vi "UHR-Fleezers Control (host) - 16.2.2v2.vi"() -> ()   [LabVIEW 2014] (continued)
                    n1840 = property on="Red Laser ON" class="Bool (strict)"("Val(Sgnl)"=TRUE ("Value (Signaling)")) -> ()  [unwired: 2 in, 2 out]
                  }
                }
              }
              frame #3 {
                n1841 = node-c288() -> (w2681:T28)  [unwired: 4 in]
                n1842 = timed-loop {
                  timing: w2681 -> [_]
                  timing-out: [_] -> w2680
                  tunnel: [w2682] -> _
                  tunnel: w2679 -> [w2682]
                  stop <- "Stop assembly line" stop-if-true
                  n1843 = node-c288() -> ()  [unwired: 1 in, 1 out]
                  n1844 = local read "APD 2 Rate (Hz)"() -> (w2686:dbl)
                  n1845 = Multiply(x="Cy5 Fl.  Thresh. (kHz)", y=1000.0) -> (x*y=w2689:dbl)
                  n1846 = Greater?(x=w2686, y=w2689) -> (0:w2685:bool)
                  n1847 = And(x=w2685, y=w2682) -> (x .and. y?=w2683:bool)
                  n1848 = case shown="True" w2683 {
                    frame False {
                    }
                    frame True {
                      n1849 = property on="Green Laser ON" class="Bool (strict)"("Val(Sgnl)"=TRUE ("Value (Signaling)")) -> ()  [unwired: 2 in, 2 out]
                    }
                  }
                  n1850 = node-c288() -> ()  [unwired: 1 in, 1 out]
                }
                n1851 = node-c288(w2680) -> ()  [unwired: 1 out]
              }
              frame #4 {
                w2696 = FALSE ("Value (Signaling)")
                # "lower spot"
                n1852 = local read "Saved Stage Positions"() -> (w2700:dbl[][])
                n1853 = property on="Red Laser ON" class="Bool (strict)"("Val(Sgnl)"=w2696) -> ()  [unwired: 2 in, 2 out]
                n1854 = property on="Green Laser ON" class="Bool (strict)"("Val(Sgnl)"=w2696) -> ()  [unwired: 2 in, 2 out]
                n1855 = local write "Stage Moving"(TRUE ("Stage Moving")) -> ()
                n1856 = local write "Stop assembly line"(FALSE ("Stop assembly line")) -> ()
                n1857 = call "move to saved stage position.vi"("Stage VISA resource name in"=w2697, "Position"=3, "Saved Stage Positions"=w2700) -> ("error out"=w2699:errorcluster)  [unwired: 1 in, 1 out]
                n1858 = local write "Stage Control Serial Error"(w2699) -> ()
              }
              frame #5 {
                w2702 = FALSE ("Stage Moving")
                n1859 = local write "Stage Moving"(w2702) -> ()
                n1860 = local write "AL Running"(w2702) -> ()
                n1861 = call <vilib>:"Beep.vi"() -> ()  [unwired: 3 in, 9 out]
              }
            }
          }
        }
      }
      event "Stop All": Value Change {
        n1862 = event-data() -> ()  [unwired: 7 out]
        n1863 = local read "Stop All"() -> (w2703:bool)
      }
    }
    n1864 = node-c288() -> ()  [unwired: 2 out]
  }
  n1865 = timed-loop "Basic control parameters (all FPGA settings, other basic controls)" {
    shift-right: [w2711] -> _
    shift-left: errorcluster {"status"=FALSE, "code"=0, "source"=""} ("error out") -> [_]
    tunnel: [w2710] -> _
    timing: w85 -> [_]
    timing-out: [_] -> w84
    tunnel: w63 -> [w2709]
    tunnel: w55 -> [w2708]
    tunnel: w54 -> [w2707]
    tunnel: w53 -> [w2706]
    tunnel: w52 -> [w2705]
    tunnel: w36 -> [w2704]
    stop <- w2710 stop-if-true
    n1866 = node-c288() -> ()  [unwired: 2 out]
    n1867 = event shown="[34] \"Read Cal\": Value Change" {
      selector: _ -> [_ _ _ _ _ _ _ _ _ _ _ _ _ _ _ _ _ _ _ _ _ _ _ _ _ _ _ _ _ _ _ _ _ _ _ _ _ _ _ _ _ _ _ _ _ _ _ _ _ _ _ _ _ _ _ _ _ _ _ _ _ _ _ _ _ _ _ _ _ _ _ _ _ _ _ _ _ _ _ _]
      dyn-events: _ -> [_ _ _ _ _ _ _ _ _ _ _ _ _ _ _ _ _ _ _ _ _ _ _ _ _ _ _ _ _ _ _ _ _ _ _ _ _ _ _ _ _ _ _ _ _ _ _ _ _ _ _ _ _ _ _ _ _ _ _ _ _ _ _ _ _ _ _ _ _ _ _ _ _ _ _ _ _ _ _ _]
      timeout: _ -> [_ _ _ _ _ _ _ _ _ _ _ _ _ _ _ _ _ _ _ _ _ _ _ _ _ _ _ _ _ _ _ _ _ _ _ _ _ _ _ _ _ _ _ _ _ _ _ _ _ _ _ _ _ _ _ _ _ _ _ _ _ _ _ _ _ _ _ _ _ _ _ _ _ _ _ _ _ _ _ _]
      tunnel: [w2754 _ _ _ w2784 _ _ _ _ _ _ w2858 _ _ w2949 w2951 w2960 w2962 w3032 _ w3074 w3101 w3129 w3154 w3181 w3207 w3238 _ _ _ w3251 w3345 w3349 w3386 _ w3424 w3427 w3430 w3440 w3443 _ w3450 _ _ _ _ _ _ _ _ _ _ _ _ _ _ _ _ _ w3914 _ _ _ _ w3950 _ _ _ _ _ _ _ _ _ _ _ _ _ _ _] -> w2711
      tunnel: [_ _ _ _ _ _ _ _ _ w2843 _ _ _ _ _ _ _ _ _ _ _ _ _ _ _ _ _ _ _ _ _ _ _ _ _ _ _ _ _ _ _ _ _ _ _ _ _ _ _ _ _ _ _ _ _ _ _ _ _ _ _ _ _ _ _ _ _ _ _ _ _ _ _ _ _ _ _ _ _ _] -> w2710
      tunnel: [_ _ _ _ _ _ _ "Round T1 X" _ _ _ _ _ _ _ _ _ _ _ _ _ _ _ _ _ _ _ _ _ _ _ _ _ _ _ _ _ _ _ _ _ _ _ _ _ _ _ _ _ _ _ _ _ _ _ _ _ _ _ _ _ _ _ _ _ _ _ _ _ _ _ _ _ _ _ _ _ _ _ _] -> _
      tunnel: [_ _ _ "Adjust Scale\nto Mean" _ _ _ _ _ _ _ _ _ _ _ _ _ _ _ _ _ _ _ _ _ _ _ _ _ _ "Test ttrig" _ _ _ _ _ _ _ _ _ _ _ _ _ _ _ _ _ _ "Flush Sample" "Flush Pump 3" "Flush Pump 1" "Clear Volume" _ _ _ _ _ _ _ _ _ _ _ _ _ _ _ _ _ _ _ _ _ _ _ _ _ _ _] -> _
      tunnel: [_ _ _ _ _ _ _ _ "Round T2 X" _ "Delayed Interlace Start" _ _ _ _ _ _ _ _ _ _ _ _ _ _ _ _ _ _ _ _ _ _ _ _ _ _ _ _ _ _ _ _ _ _ _ _ _ _ _ _ _ _ _ _ _ _ _ _ _ _ _ _ _ _ _ _ _ _ _ _ _ _ _ _ _ _ _ _ _] -> _
      tunnel: w2709 -> [_ _ _ _ _ _ _ _ _ _ _ _ _ _ _ _ _ _ _ _ _ _ _ _ _ _ _ _ _ _ _ _ _ _ _ _ _ _ _ _ _ _ _ _ _ w3649 w3656 w3663 w3668 w3682 _ _ w3828 _ _ _ _ _ _ _ _ _ _ _ _ _ _ _ _ _ _ _ _ _ _ _ _ _ _ _]
      tunnel: w2708 -> [_ _ _ _ _ _ _ _ _ _ _ _ _ _ _ _ _ _ _ _ _ _ _ _ _ _ _ _ _ _ _ _ _ _ _ _ _ _ _ _ _ _ _ w3538 _ _ _ _ _ _ w3741 _ _ w3834 _ w3843 _ w3857 _ _ _ _ _ _ _ _ _ _ _ _ _ _ _ _ _ _ _ _ _ _]
      tunnel: w2707 -> [_ _ _ _ _ _ _ _ _ _ _ _ _ _ _ _ _ _ _ _ _ _ _ _ _ _ _ _ _ _ _ _ _ _ _ _ _ _ _ _ _ _ _ _ _ _ _ _ _ _ _ _ _ _ _ _ _ _ _ _ _ _ _ _ _ _ _ _ _ _ _ _ _ _ _ _ _ _ _ _]
      tunnel: w2706 -> [_ _ _ _ _ _ _ _ _ _ _ _ _ _ _ _ _ _ _ _ _ _ _ _ _ _ _ _ _ _ _ _ _ _ _ _ _ _ _ _ _ _ w3461 _ _ _ _ _ _ _ _ w3786 _ _ w3839 _ w3850 _ w3882 _ _ _ _ _ _ _ _ _ _ _ _ _ _ _ _ _ _ _ _ _]
      tunnel: w2705 -> [_ _ _ _ _ _ _ _ _ _ _ _ _ _ _ _ _ _ _ _ _ _ _ _ _ _ _ _ _ _ _ _ _ _ _ _ _ _ _ _ _ _ _ _ _ _ _ _ _ _ _ _ _ _ _ _ _ _ _ _ _ _ _ _ _ _ _ _ _ _ _ _ _ _ _ _ _ _ _ _]
      tunnel: w2704 -> [w2718 _ _ _ w2783 _ w2809 _ _ _ _ w2849 _ _ w2931 w2950 w2955 w2961 w2997 _ w3063 w3099 w3115 w3136 w3164 w3184 w3216 w3242 w3246 w3247 w3249 w3253 w3346 w3351 _ w3421 w3425 w3428 w3438 w3441 _ w3449 _ _ _ _ _ _ _ _ _ _ _ _ _ _ _ _ _ w3907 _ w3928 _ w3934 w3949 _ w3956 w3958 w3965 w3979 w3994 _ w4003 _ w4023 _ _ w4079 w4115 w4116]
      event "AI Count (ticks)", "Sets to FIFO (Traps)", "Save ave N", "FPGA Ave.", "# Samples/channel", "N sets to save", "APD Samples/FIFO Acq.": Value Change {
        # "So that if 'Save ave N' is updated, the AOD scanning code updates too."
        n1868 = event-data() -> ()  [unwired: 6 out]
        n1869 = local read "AI Count (ticks)"() -> (w2738:u16)
        n1870 = Unbundle By Name("Sets to FIFO (Traps)") -> ("Set 1"=w2722:bool, "Set 2"=w2721:bool, "Set 3"=w2720:bool)
        n1871 = Boolean To (0,1)(Boolean="Sets to FIFO (Traps)") -> (0, 1=w2746:cluster{"Set 1":i16, "Set 2":i16, "Set 3":i16})
        n1872 = xnode "Read/Write Control"("FPGA VI Reference In"=w2718, "ai count"=w2738, "Set 1"=w2722, "Set 2"=w2721, "Set 3"=w2720, "N of AI1 Int Acq Sets"="N Acq Sets (Traps + Fl.)") -> ("error out"=w2754:errorcluster)  [unwired: 1 in, 1 out]
        n1873 = Cluster To Array(cluster=w2746) -> (array=w2745:i16[])
        n1874 = To Unsigned Long Integer(number=w2745) -> (unsigned 32bit integer=w2727:u32[])
        n1875 = local read "Scan steps (AOD)"() -> (w2747:u64)
        n1876 = Multiply(x=w2738, y="N Acq Sets (Traps + Fl.)") -> (x*y=w2736:u16)
        n1877 = Divide(x=40000000.0, y=w2738) -> (x/y=w2730:dbl)
        "AI rate (Hz)" <- w2730
        "Ave. Rate (Hz)" <- w2730
        n1878 = Add Array Elements(numeric array=w2727) -> (sum=w2739:u32)
        "Trap Sets" <- w2739
        n1879 = Reciprocal(x=w2730) -> (1/x=→"Ave. Period (s)":dbl)
        n1880 = property on="Scan steps (AOD)" class="DigNum (strict)"("Val(Sgnl)"=w2747) -> ()  [unwired: 2 in, 2 out]
        n1881 = Divide(x=w2730, y="N Acq Sets (Traps + Fl.)") -> (x/y=w2751:dbl)
        "Data Rate (Hz)" <- w2751
        n1882 = Reciprocal(x=w2751) -> (1/x=→"Data Period (s)":dbl)
        n1883 = local read "Save ave N"() -> (w2750:dbl)
        n1884 = Divide(x=w2751, y=w2750) -> (x/y=w2749:dbl)
        "Save Data Rate (Hz)" <- w2749
        n1885 = Reciprocal(x=w2749) -> (1/x=→"Save Data Period (s)":dbl)
        n1886 = Multiply(x=w2736, y="# Samples/trap") -> (x*y=w2734:u32)
        "Counts/DMA" <- w2734
        n1887 = property on="Trap Disp. Downsample" class="DigNum (strict)"("Maximum"="# Samples/trap") -> ()  [unwired: 2 in, 2 out]
        n1888 = Multiply(x=w2739, y="# Samples/trap") -> (x*y=w2728:u32)
        "# Samples/channel" <- w2728
        n1889 = Multiply(x=w2728, y=u32 8) -> (x*y=→"Trap AI Elements/DMA read":u32)
        n1890 = local read "APD Int. Count"() -> (w2735:u32)
        n1891 = Multiply(x=w2728, y=u32 3) -> (x*y=→"Trap Pos Elements/DMA read":u32)
        n1892 = Divide(x=w2734, y=w2735) -> (x/y=w2717:dbl)
        "APD Samples/FIFO Acq." <- w2717
        n1893 = Divide(x=w2734, y=40000000.0) -> (x/y=w2732:dbl)
        "DMA Update Period (s)" <- w2732
        n1894 = local read "Number of APDs"() -> (w2719:u8)
        n1895 = Multiply(x=w2719, y=w2717) -> (x*y=→"APD Elements/DMA read":dbl)
        n1896 = property on="APD Disp. Downsample" class="DigNum (strict)"("Maximum"=w2717) -> ()  [unwired: 2 in, 2 out]
        n1897 = Quotient & Remainder(x=w2717, y=1.0) -> (x-y*floor(x/y)=w2715:dbl)  [unwired: 1 out]
        n1898 = Equal To 0?(x=w2715) -> (x = 0?=→"Integer?":bool)
        n1899 = local read "N sets to save"() -> (w2744:u32)
        n1900 = Multiply(x=w2732, y=w2744) -> (x*y=→"Total Time (s)":dbl)
        "FPGA Averaging" <- FALSE ("FPGA Averaging")
      }
      event "Remove Offset": Value Change {
        n1901 = event-data() -> ()  [unwired: 7 out]
        n1902 = local write "Remove Offset"(FALSE ("Remove Offset")) -> ()
        n1903 = local read "Bead Mean (nm)"() -> (w2756:dbl)
        n1904 = local read "Offset (nm)"() -> (w2757:dbl)
        n1905 = Add(x=w2756, y=w2757) -> (x+y=w2755:dbl)
        n1906 = local write "Offset (nm)"(w2755) -> ()
        n1907 = disable-structure shown="Disabled" {
          frame Disabled {
            n1908 = local read "Bead Mean (nm)"() -> (w2762:dbl)
            n1909 = Add(y=w2762) -> (x=w2761:dbl, x+y=w2760:dbl)
            n1910 = Subtract(x=w2762, y=w2761) -> (x-y=w2759:dbl)
            n1911 = property on="Bead Separation" class="WFChart (strict)"("YScale.Minimum"=w2759) -> ()  [unwired: 2 in, 2 out]
            n1912 = property on="Bead Separation" class="WFChart (strict)"("YScale.Maximum"=w2760) -> ()  [unwired: 2 in, 2 out]
          }
          frame Enabled {
          }
        }
      }
      event "Detector Type": Value Change {
        n1913 = event-data() -> ()  [unwired: 7 out]
        n1914 = local read "AI labels"() -> (w2764:string[])
        n1915 = property on="High Res. Display" class="Ring (strict)"("Strings []"=w2764) -> ()  [unwired: 2 in, 2 out]
        n1916 = Build Array (concatenate)(w2764, "none") -> (w2765:string[])
        n1917 = property on="FFT 1 Choice 1" class="Ring (strict)"("Strings []"=w2765) -> ()  [unwired: 2 in, 2 out]
        n1918 = property on="FFT 1 Choice 2" class="Ring (strict)"("Strings []"=w2765) -> ()  [unwired: 2 in, 2 out]
        n1919 = property on="FFT 2 Choice 1" class="Ring (strict)"("Strings []"=w2765) -> ()  [unwired: 2 in, 2 out]
        n1920 = property on="FFT 2 Choice 2" class="Ring (strict)"("Strings []"=w2765) -> ()  [unwired: 2 in, 2 out]
        n1921 = Bundle("APD 1", "APD 2", "APD 3") -> (w2768:cluster{string, string, string})  [unwired: 1 out]
        n1922 = Cluster To Array(cluster=w2768) -> (array=w2766:string[])
        n1923 = Build Array (concatenate)(w2766, w2765) -> (w2770:string[])
        n1924 = Array Size(array=w2770) -> (size(s)=w2771:i32)
        n1925 = property on="Signals to Plot" class="LstBox (strict)"("Item Names"=w2770) -> ()  [unwired: 2 in, 2 out]
        n1926 = property on="Signals to Plot" class="LstBox (strict)"("Number of Rows"=w2771) -> ()  [unwired: 2 in, 2 out]
        n1927 = property on="All Signals" class="WFChart (strict)"("LegNumRows"=w2771) -> ()  [unwired: 2 in, 2 out]
      }
      event "Adjust Scale\nto Mean": Value Change {
        n1928 = event-data() -> ()  [unwired: 7 out]
        n1929 = local read "APD 1 Rate (Hz)"() -> (w2780:dbl)
        n1930 = Multiply(x=1000.0, y="Above (kHz)") -> (x*y=w2778:dbl)
        n1931 = Multiply(x=1000.0, y="Below (kHz)") -> (x*y=w2776:dbl)
        n1932 = Add(x=w2778, y=w2780) -> (x+y=w2773:dbl)
        n1933 = Subtract(x=w2780, y=w2776) -> (x-y=w2774:dbl)
        n1934 = property on="APD Chart" class="WFChart (strict)"("YScale.Minimum"=w2774) -> ()  [unwired: 2 in, 2 out]
        n1935 = property on="APD Chart" class="WFChart (strict)"("YScale.Maximum"=w2773) -> ()  [unwired: 2 in, 2 out]
      }
      event "Phase adj. (AI1)", "+ phase (AI1)", "- phase (AI1)": Value Change {
        n1936 = event-data() -> ()  [unwired: 7 out]
        n1937 = Negate(x="Phase adj. (AI1)") -> (-x=w2791:i16)
        n1938 = Select(t=w2791, s="- phase (AI1)", f="Phase adj. (AI1)") -> (s? t:f=w2790:i16)
        n1939 = xnode "Read/Write Control"("FPGA VI Reference In"=w2783, "Phase count adjustment"=w2790) -> ("FPGA VI Reference Out"=w2789:T25, "error out"=w2788:errorcluster)  [unwired: 2 in]
        n1940 = Or(x="- phase (AI1)", y="+ phase (AI1)") -> (x .or. y?=w2785:bool)
        n1941 = xnode "Read/Write Control"("FPGA VI Reference In"=w2789, "error in"=w2788, "+ phase"=w2785) -> ("error out"=w2784:errorcluster)  [unwired: 1 in, 1 out]
      }
      event "Signals to Plot": Double Click {
        w2795 = u32 9868950 ("Color Box")
        n1942 = event-data() -> ("Row"=w2797:i32)  [unwired: 9 out]
        n1943 = property on="All Signals" class="WFChart (strict)"("Active Plot"=w2797) -> (error out=w2808:errorcluster)  [unwired: 2 in, 1 out]
        n1944 = property on="All Signals" class="WFChart (strict)" props=["Plot", "Visible?", "Plot", "Plot Color"](error in=w2808) -> (error out=w2807:errorcluster, "Plot.Visible?"=w2806:bool)  [unwired: 1 in, 2 out]
        n1945 = Select(t=FALSE ("Plot.Visible"), s=w2806, f=TRUE ("Plot.Visible")) -> (s? t:f=w2801:bool)
        n1946 = property on="All Signals" class="WFChart (strict)"(error in=w2807, "Plot.Visible?"=w2801) -> (error out=w2803:errorcluster)  [unwired: 1 in, 1 out]
        n1947 = property on="All Signals" class="WFChart (strict)"(error in=w2803) -> (error out=w2798:errorcluster, "Plot.Plot Color"=w2802:u32)  [unwired: 1 in, 1 out]
        n1948 = property on="Signals to Plot" class="LstBox (strict)"(error in=w2798, "Active Row"=w2797) -> (error out=w2796:errorcluster)  [unwired: 1 in, 1 out]
        n1949 = Select(t=w2802, s=w2801, f=u32 0) -> (s? t:f=w2799:u32)
        n1950 = property on="Signals to Plot" class="LstBox (strict)"(error in=w2796, "CellFontColor"=w2799, "SelColor"=w2795, "CellBG"=w2795, "CellFontSize"=u32 20 ("Active Row:Cell Font:Size"), "CellFontBold"=TRUE ("Active Row:Cell Font:Bold")) -> ()  [unwired: 1 in, 2 out]
      }
      event "BD 1 Frequency 1 (MHz)", "BD 1 Frequency 2 (MHz)", "BD 1 Frequency 3 (MHz)", "BD 2 Frequency 1 (MHz)", "BD 2 Frequency 2 (MHz)", "BD 2 Frequency 3 (MHz)", "Trap Delta (MHz)", "Update all trap values": Value Change {
        # "This is so you can set trap frequencies\nvia local variables and then update\nall at once"
        n1951 = event-data() -> ("CtlRef"=w2813:refnum<vi>)  [unwired: 6 out]
        n1952 = control-ref of="Trap Delta (MHz)"() -> (w2812:refnum<vi>)
        n1953 = Equal?(x=w2812, y=w2813) -> (x = y?=w2811:bool)
        n1954 = local write "Update all trap values"(FALSE ("Update all trap values")) -> ()
        n1955 = case shown="False" "Oscillate Set 1" {
          tunnel: w2811 -> [w2821 _]
          tunnel: w2809 -> [w2819 _]
          frame False {
            n1956 = local read "BD 1 Frequency 2 (MHz)"() -> (w2825:dbl)
            n1957 = local read "BD 1 Frequency 1 (MHz)"() -> (w2823:dbl)
            n1958 = Subtract(x=w2825, y="Trap Delta (MHz)") -> (x-y=w2822:dbl)
            n1959 = Select(t=w2822, s=w2821, f=w2823) -> (s? t:f=w2820:dbl)
            n1960 = local read "Y RF Frequency Limits (MHz)"() -> (w2826:T18)
            n1961 = local read "X RF Frequency Limits (MHz)"() -> (w2827:T18)
            n1962 = local write "BD 1 Frequency 1 (MHz)"(w2820) -> ()
            n1963 = local read "BD 1 Frequency 3 (MHz)"() -> (w2835:dbl)
            n1964 = local read "BD 2 Frequency 1 (MHz)"() -> (w2830:dbl)
            n1965 = local read "BD 2 Frequency 2 (MHz)"() -> (w2829:dbl)
            n1966 = local read "BD 2 Frequency 3 (MHz)"() -> (w2836:dbl)
            n1967 = call "set RF board frequency - interlace.vi"("Board 2 Frequency Limits"=w2826, "Board 1 Frequency Limits"=w2827, "FPGA VI Reference In"=w2819, "Board 2 Frequency 3 (MHz)"=w2836, "Board 1 Frequency 3 (MHz)"=w2835, "Board 2 Frequency 2 (MHz)"=w2829, "Board 2 Frequency 1 (MHz)"=w2830, "Board 1 Frequency 2 (MHz)"=w2825, "Board 1 Frequency 1  (MHz)"=w2820) -> ()  [unwired: 1 in, 2 out]
            n1968 = Subtract(x=w2830, y=w2829) -> (x-y=w2833:dbl)
            n1969 = Subtract(x=w2820, y=w2825) -> (x-y=w2834:dbl)
            n1970 = Square(x=w2833) -> (x^2=w2817:dbl)
            n1971 = Square(x=w2834) -> (x^2=w2832:dbl)
            n1972 = Select(t=0.0, s="Ignore BD 2 for trap delta", f=w2817) -> (s? t:f=w2816:dbl)
            n1973 = Add(x=w2832, y=w2816) -> (x+y=w2831:dbl)
            n1974 = Square Root(x=w2831) -> (sqrt(x)=w2828:dbl)
            n1975 = property on="Initial delta (MHz)" class="DigNum (strict)"("Val(Sgnl)"=w2828) -> ()  [unwired: 2 in, 2 out]
            n1976 = local write "Trap Delta (MHz)"(w2828) -> ()
          }
          frame True {
          }
        }
      }
      event "Round T1 X": Value Change {
        n1977 = event-data() -> ()  [unwired: 7 out]
        n1978 = local read "BD 1 Frequency 1 (MHz)"() -> (w2839:dbl)
        n1979 = Round To Nearest(number=w2839) -> (nearest integer value=w2838:dbl)
        n1980 = property on="BD 1 Frequency 1 (MHz)" class="DigNum (strict)"("Val(Sgnl)"=w2838) -> ()  [unwired: 2 in, 2 out]
      }
      event "Round T2 X": Value Change {
        n1981 = event-data() -> ()  [unwired: 7 out]
        n1982 = local read "BD 1 Frequency 2 (MHz)"() -> (w2841:dbl)
        n1983 = Round To Nearest(number=w2841) -> (nearest integer value=w2840:dbl)
        n1984 = property on="BD 1 Frequency 2 (MHz)" class="DigNum (strict)"("Val(Sgnl)"=w2840) -> ()  [unwired: 2 in, 2 out]
      }
      event "Stop All": Value Change {
        n1985 = event-data() -> ()  [unwired: 7 out]
        n1986 = local read "Stop All"() -> (w2843:bool)
      }
      event "Delayed Interlace Start": Value Change {
        n1987 = event-data() -> ()  [unwired: 7 out]
        n1988 = flat-sequence {
          frame #0 {
            n1989 = Multiply(x="Delay to Interlace (s)", y=1000.0) -> (x*y=w2845:dbl)
            n1990 = Wait (ms)(milliseconds to wait=w2845) -> ()  [unwired: 1 out]
          }
          frame #1 {
            n1991 = property on="Laser interlacing mode" class="RadioBtnsControl (strict)"("Val(Sgnl)"=enum32{"Laser ON", "Laser OFF", "Interlace"}."Interlace" ("Value (Signaling)")) -> ()  [unwired: 2 in, 2 out]
          }
        }
      }
      event "BD 1 Amplitude 1 (%)", "BD 1 Amplitude 2 (%)", "BD 1 Amplitude 3 (%)", "BD 2 Amplitude 1 (%)", "BD 2 Amplitude 2 (%)", "BD 2 Amplitude 3 (%)", "Trap 1 ON", "Trap 2 ON", "Trap 3 ON", "Feedback On/Off", "All FB On/Off": Value Change {
        w2870 = i16 1 ("f")
        n1992 = event-data() -> ()  [unwired: 7 out]
        n1993 = local write "Trap 1 (ON/OFF)"("Trap 1 ON") -> ()
        n1994 = local write "Trap 2 (ON/OFF)"("Trap 2 ON") -> ()
        n1995 = Boolean To (0,1)(Boolean="Trap 3 ON") -> (0, 1=w2871:i16)
        n1996 = Boolean To (0,1)(Boolean="Trap 1 ON") -> (0, 1=w2872:i16)
        n1997 = Boolean To (0,1)(Boolean="Trap 2 ON") -> (0, 1=w2873:i16)
        n1998 = Select(t=w2873, s="Trap ON/OFF X or Y Amp?", f=w2870) -> (s? t:f=w2868:i16)
        n1999 = Select(t=w2872, s="Trap ON/OFF X or Y Amp?", f=w2870) -> (s? t:f=w2869:i16)
        n2000 = Select(t=w2871, s="Trap ON/OFF X or Y Amp?", f=w2870) -> (s? t:f=w2867:i16)
        n2001 = Select(t=w2870, s="Trap ON/OFF X or Y Amp?", f=w2873) -> (s? t:f=w2865:i16)
        n2002 = Select(t=w2870, s="Trap ON/OFF X or Y Amp?", f=w2872) -> (s? t:f=w2866:i16)
        n2003 = Select(t=w2870, s="Trap ON/OFF X or Y Amp?", f=w2871) -> (s? t:f=w2864:i16)
        n2004 = And(x="All FB On/Off", y="Feedback On/Off") -> (x .and. y?=w2862:cluster{"Set 1":bool, "Set 2":bool})
        n2005 = local read "BD 1 Amplitude 1 (%)"() -> (w2880:dbl)
        n2006 = local read "BD 1 Amplitude 2 (%)"() -> (w2879:dbl)
        n2007 = local read "BD 1 Amplitude 3 (%)"() -> (w2878:dbl)
        n2008 = Unbundle By Name(w2862) -> ("Set 1"=w2857:bool, "Set 2"=w2854:bool)
        n2009 = local read "Y RF Amplitude Limits (%)"() -> (w2850:T18)
        n2010 = local read "X RF Amplitude Limits (%)"() -> (w2851:T18)
        n2011 = local read "BD 2 Amplitude 1 (%)"() -> (w2881:dbl)
        n2012 = local read "BD 2 Amplitude 2 (%)"() -> (w2882:dbl)
        n2013 = local read "BD 2 Amplitude 3 (%)"() -> (w2883:dbl)
        n2014 = And(x="Trap 2 ON", y=w2854) -> (x .and. y?=w2852:bool)
        n2015 = And(x="Trap 1 ON", y=w2857) -> (x .and. y?=w2855:bool)
        n2016 = Multiply(x=w2869, y=w2880) -> (x*y=w2877:dbl)
        n2017 = Multiply(x=w2879, y=w2868) -> (x*y=w2875:dbl)
        n2018 = Multiply(x=w2878, y=w2867) -> (x*y=w2876:dbl)
        n2019 = Multiply(x=w2881, y=w2866) -> (x*y=w2884:dbl)
        n2020 = Multiply(x=w2882, y=w2865) -> (x*y=w2885:dbl)
        n2021 = Multiply(x=w2883, y=w2864) -> (x*y=w2886:dbl)
        n2022 = call "set RF board amplitude - interlace.vi"("Board 2 Amplitude Limits"=w2850, "Board 1 Amplitude Limits"=w2851, "FPGA VI Reference In"=w2849, "Board 2 Amplitude 3 (%)"=w2886, "Board 1 Amplitude 3 (%)"=w2876, "Board 2 Amplitude 2 (%)"=w2885, "Board 2 Amplitude 1 (%)"=w2884, "Board 1 Amplitude 2 (%)"=w2875, "Board 1 Amplitude 1 (%)"=w2877) -> ("error out"=w2859:errorcluster, "FPGA VI Reference Out"=w2860:T25)  [unwired: 1 in]
        n2023 = xnode "Read/Write Control"("FPGA VI Reference In"=w2860, "error in"=w2859, "FB On/Off Set 1"=w2855, "FB On/Off Set 2"=w2852) -> ("error out"=w2858:errorcluster)  [unwired: 1 out]
      }
      event "Load parameters": Value Change {
        n2024 = event-data() -> ()  [unwired: 7 out]
        n2025 = property on="Saved AOD Raster Scan Parameter Sets" class="Arr (strict)"() -> ("Index Values"=w2897:u32[])  [unwired: 2 in, 2 out]
        n2026 = Index Array(array=w2897, index=0) -> (element=w2894:u32)
        n2027 = local write "Load parameters"(FALSE ("Load parameters")) -> ()
        n2028 = Index Array(array="Saved AOD Raster Scan Parameter Sets", index=w2894) -> (element=w2893:T38)
        n2029 = Unbundle By Name(w2893) -> ("Scan Range AOD (nm) 2"=w2892:dbl, "Step Size AOD (nm) 2"=w2891:dbl, "Scan Speed AOD (nm/s) 2"=w2890:dbl, "Number of scans (AOD) 2"=w2889:u16)
        n2030 = flat-sequence {
          tunnel: w2892 -> [w2900]
          tunnel: w2891 -> [w2899]
          tunnel: w2890 -> [w2898]
          tunnel: w2889 -> [w2901]
          frame #0 {
            n2031 = local write "Scan Speed (nm/s)"(w2898) -> ()
            n2032 = local write "Scan Range (nm)"(w2900) -> ()
            n2033 = local write "Step Size (nm)"(w2899) -> ()
          }
          frame #1 {
            n2034 = property on="Number of F/B Scans (AOD)" class="DigNum (strict)"("Val(Sgnl)"=w2901) -> ()  [unwired: 2 in, 2 out]
          }
        }
      }
      event "Trap 1 (ON/OFF)", "Trap 2 (ON/OFF)": Value Change {
        n2035 = event-data() -> ()  [unwired: 7 out]
        n2036 = flat-sequence {
          tunnel: [w2911] -> w2906
          tunnel: w2906 -> [w2926]
          tunnel: [w2912] -> w2902
          frame #0 {
            n2037 = local read "Trap 1 ON"() -> (w2911:bool)
          }
          frame #1 {
            n2038 = Exclusive Or(1:w2926, 2:"Trap 1 (ON/OFF)") -> (0:w2919:bool)
            n2039 = Select(t="on", s="Trap 2 (ON/OFF)", f="off") -> (s? t:f=w2918:string)
            n2040 = Select(t="on", s="Trap 1 (ON/OFF)", f="off") -> (s? t:f=w2914:string)
            n2041 = Build Array("trap 1 ", w2914) -> (w2913:string[])
            n2042 = Build Array("trap 2 " ("f"), w2918) -> (w2916:string[])
            n2043 = Select(t=w2913, s=w2919, f=w2916) -> (s? t:f=w2912:string[])
            n2044 = property on="Trap 1 ON" class="Bool (strict)"("Val(Sgnl)"="Trap 1 (ON/OFF)") -> ()  [unwired: 2 in, 2 out]
            n2045 = property on="Trap 2 ON" class="Bool (strict)"("Val(Sgnl)"="Trap 2 (ON/OFF)") -> ()  [unwired: 2 in, 2 out]
          }
        }
        n2046 = local read "Saving..."() -> (w2905:bool)
        n2047 = local read "Save Event Log?"() -> (w2904:bool)
        n2048 = And(x=w2905, y=w2904) -> (x .and. y?=w2903:bool)
        n2049 = case shown="True" w2903 {
          tunnel: w2902 -> [_ w2910]
          frame False {
          }
          frame True {
            n2050 = local read "Time (s)"() -> (w2907:dbl)
            n2051 = local read "log file ref"() -> (w2909:refnum<file>)
            n2052 = Concatenate Strings(w2910) -> (w2908:string)
            n2053 = call "write to event log.vi"("log file ref"=w2909, "time"=w2907, "input string"=w2908) -> ()  [unwired: 8 in]
          }
        }
      }
      event "DIO count 1 (ticks)", "DIO count 2 (ticks)", "DIO count 3 (ticks)", "Interlace", "Number Interlace Sets", "Not-Interlacing Set", "BD 1 Delay (ticks)", "BD 2 Delay (Ticks)", "Next trap write delay (ticks)", "Phase offset method", "Phase Increment Trap 1", "RF phase reset before cycles", "Phase Increment Trap 2": Value Change {
        n2054 = event-data() -> ()  [unwired: 7 out]
        n2055 = local read "RF phase reset before cycles"() -> (w2929:bool)
        n2056 = local read "Phase offset method"() -> (w2930:u8)
        n2057 = local read "Phase Increment Trap 1"() -> (w2928:fxp<+,14,14>)
        n2058 = local read "DIO count 3 (ticks)"() -> (w2945:u16)
        n2059 = local read "DIO count 1 (ticks)"() -> (w2947:u16)
        n2060 = local read "DIO count 2 (ticks)"() -> (w2946:u16)
        n2061 = To Unsigned Byte Integer(number="Not-Interlacing Set") -> (unsigned 8bit integer=w2936:u8)
        n2062 = Add(x=w2936, y=u8 1) -> (x+y=w2940:u8)
        n2063 = Build Array(w2947, w2946, w2945) -> (w2938:u16[])
        n2064 = Split 1D Array(array=w2938, index="Number Interlace Sets") -> (first subarray=w2948:u16[])  [unwired: 1 out]
        n2065 = xnode "Read/Write Control"("FPGA VI Reference In"=w2931, "DIO count 1 (ticks)"=w2947, "DIO count 2 (ticks)"=w2946, "DIO count 3 (ticks)"=w2945, "Interlace ON/OFF"="Interlace", "Number Interlace Cycles"="Number Interlace Sets", "Interlace Off Parameters"=w2940, "BD 1 Delay (ticks)"="BD 1 Delay (ticks)", "BD 2 Delay (Ticks)"="BD 2 Delay (Ticks)", "Next trap write delay (ticks)"="Next trap write delay (ticks)", "Phase offset method"=w2930, "RF phase reset before cycles"=w2929, "Phase Trap 1"=w2928, "Phase Trap 2"="Phase Increment Trap 2") -> ("error out"=w2949:errorcluster)  [unwired: 1 in, 1 out]
        n2066 = Index Array(array=w2938, index=w2936) -> (element=w2937:u16)
        n2067 = Add Array Elements(numeric array=w2948) -> (sum=w2942:u16)
        n2068 = Select(t=w2942, s="Interlace", f=w2937) -> (s? t:f=→"Total Counts (ticks)":u16)
      }
      event "Reset Feedback": Value Change {
        n2069 = event-data() -> ()  [unwired: 7 out]
        n2070 = Unbundle By Name("Reset Feedback") -> ("Set 1"=w2953:bool, "Set 2"=w2952:bool)
        n2071 = xnode "Read/Write Control"("FPGA VI Reference In"=w2950, "FB Reset Set 1"=w2953, "FB Reset Set 2"=w2952) -> ("error out"=w2951:errorcluster)  [unwired: 1 in, 1 out]
      }
      event "Trap Intensity PID Gains": Value Change {
        n2072 = event-data() -> ()  [unwired: 7 out]
        n2073 = Unbundle By Name("Trap Intensity PID Gains") -> ("proportional gain (Kc)"=w2958:i16, "integral gain (Kc*Ts/Ti)"=w2957:i16, "derivative gain (Kc*Td/Ts)"=w2956:i16)
        n2074 = xnode "Read/Write Control"("FPGA VI Reference In"=w2955, "P1"=w2958, "I1"=w2957, "D1"=w2956) -> ("error out"=w2960:errorcluster)  [unwired: 1 in, 1 out]
      }
      event "AI2 to Setpoint", "Setpoints (V)": Value Change {
        n2075 = event-data() -> ()  [unwired: 7 out]
        n2076 = xnode "Read/Write Control"("FPGA VI Reference In"=w2961) -> ("FPGA VI Reference Out"=w2964:T25, "error out"=w2963:errorcluster, "AI2 Y Sum Set 1"=w2971:i16, "AI2 Y Sum Set 2"=w2970:i16)  [unwired: 1 in]
        n2077 = Cluster To Array(cluster="AI2 to Setpoint") -> (array=w2974:bool[])
        n2078 = local read "AI2 (V)"() -> (w2972:cluster{"Set 1":dbl, "Set 2":dbl})
        n2079 = Or Array Elements(Boolean array=w2974) -> (logical OR=w2975:bool)
        n2080 = Bundle By Name(cluster=w2972, "Set 1"=w2971, "Set 2"=w2970) -> (w2969:cluster{"Set 1":dbl, "Set 2":dbl})
        n2081 = Divide(x=w2969, y=3276.7) -> (x/y=w2968:cluster{"Set 1":dbl, "Set 2":dbl})
        "AI2 (V)" <- w2968
        n2082 = case shown="True" w2975 {
          tunnel: [w2978 w2995] -> w2967
          tunnel: "AI2 to Setpoint" -> [_ w2991]
          tunnel: "Setpoints (V)" -> [w2979 w2994]
          tunnel: w2968 -> [_ w2988]
          frame False {
            n2083 = Multiply(x=3276.7, y=w2979) -> (x*y=w2980:cluster{"Set 1":dbl, "Set 2":dbl})
            n2084 = To Word Integer(number=w2980) -> (16bit integer=w2978:cluster{"Set 1":i16, "Set 2":i16})
          }
          frame True {
            n2085 = Unbundle By Name(w2988) -> ("Set 1"=w2987:dbl, "Set 2"=w2986:dbl)
            n2086 = Unbundle By Name(w2994) -> ("Set 1"=w2993:dbl, "Set 2"=w2992:dbl)
            n2087 = Unbundle By Name(w2991) -> ("Set 1"=w2990:bool, "Set 2"=w2989:bool)
            n2088 = Select(t=w2987, s=w2990, f=w2993) -> (s? t:f=w2985:dbl)
            n2089 = Select(t=w2986, s=w2989, f=w2992) -> (s? t:f=w2984:dbl)
            n2090 = Bundle By Name(cluster=w2994, "Set 1"=w2985, "Set 2"=w2984) -> (w2982:cluster{"Set 1":dbl, "Set 2":dbl})
            n2091 = local write "Setpoints (V)"(w2982) -> ()
            n2092 = Multiply(x=3276.7, y=w2982) -> (x*y=w2983:cluster{"Set 1":dbl, "Set 2":dbl})
            n2093 = To Word Integer(number=w2983) -> (16bit integer=w2995:cluster{"Set 1":i16, "Set 2":i16})
          }
        }
        n2094 = Unbundle By Name(w2967) -> ("Set 1"=w2966:i16, "Set 2"=w2965:i16)
        n2095 = xnode "Read/Write Control"("FPGA VI Reference In"=w2964, "error in"=w2963, "FB Setpoint Set 1"=w2966, "FB Setpoint Set 2"=w2965) -> ("error out"=w2962:errorcluster)  [unwired: 1 out]
      }
      event "+ phase (GI)", "- phase (GI)", "+ phase (GI) 2", "- phase (GI) 2", "+ phase (RI)", "- phase (RI)", "+ phase (Green FB)", "- phase (Green FB)", "- phase (BI AO)", "+ phase (BI AO)", "- phase (BI DO)", "+ phase (BI DO)": Value Change {
        n2096 = event-data() -> ()  [unwired: 7 out]
        n2097 = Or(x="+ phase (GI)", y="- phase (GI)") -> (x .or. y?=w3031:bool)
        n2098 = Negate(x="Phase adj. (GI)") -> (-x=w3036:i16)
        n2099 = Select(t=w3036, s="+ phase (GI)", f="Phase adj. (GI)") -> (s? t:f=w3035:i16)
        n2100 = Or(x="+ phase (GI) 2", y="- phase (GI) 2") -> (x .or. y?=w3022:bool)
        n2101 = Negate(x="Phase adj. (GI) 2") -> (-x=w3027:i16)
        n2102 = Select(t=w3027, s="+ phase (GI) 2", f="Phase adj. (GI) 2") -> (s? t:f=w3023:i16)
        n2103 = Negate(x="Phase adj. (RI)") -> (-x=w3021:i16)
        n2104 = Or(x="+ phase (RI)", y="- phase (RI)") -> (x .or. y?=w3017:bool)
        n2105 = Select(t=w3021, s="+ phase (RI)", f="Phase adj. (RI)") -> (s? t:f=w3016:i16)
        n2106 = Or(x="+ phase (Green FB)", y="- phase (Green FB)") -> (x .or. y?=w3010:bool)
        n2107 = Negate(x="Phase adj. (Green FB)") -> (-x=w3015:i16)
        n2108 = Select(t=w3015, s="+ phase (Green FB)", f="Phase adj. (Green FB)") -> (s? t:f=w3011:i16)
        n2109 = Negate(x="Phase adj. (BI AO)") -> (-x=w3009:i16)
        n2110 = Or(x="+ phase (BI AO)", y="- phase (BI AO)") -> (x .or. y?=w2999:bool)
        n2111 = Select(t=w3009, s="+ phase (BI AO)", f="Phase adj. (BI AO)") -> (s? t:f=w3001:i16)
        n2112 = Negate(x="Phase adj. (BI DO)") -> (-x=w3005:i16)
        n2113 = Or(x="+ phase (BI DO)", y="- phase (BI DO)") -> (x .or. y?=w2998:bool)
        n2114 = Select(t=w3005, s="+ phase (BI DO)", f="Phase adj. (BI DO)") -> (s? t:f=w3000:i16)
        n2115 = xnode "Read/Write Control"("FPGA VI Reference In"=w2997, "Phase count adjustment (GI)"=w3035, "Phase count adjustment (GI) 2"=w3023, "Phase count adjustment (RI)"=w3016, "Phase count adjustment (Green FB)"=w3011, "Phase count adjustment (BI AO)"=w3001, "Phase count adjustment (BI D)"=w3000) -> ("FPGA VI Reference Out"=w3033:T25, "error out"=w3034:errorcluster)  [unwired: 1 in]
        n2116 = xnode "Read/Write Control"("FPGA VI Reference In"=w3033, "error in"=w3034, "+ phase (GI)"=w3031, "+ phase (GI) 2"=w3022, "+ phase (RI)"=w3017, "+ phase (Green FB)"=w3010, "+ phase (BI AO)"=w2999, "+ phase (BI D)"=w2998) -> ("error out"=w3032:errorcluster)  [unwired: 1 out]
      }
      event "Green Laser ON/OFF", "Red Laser ON/OFF", "Blue Laser ON/OFF": Value Change {
        # "This loop shouldn't be initialized.  The main 'laser ON' settings should dominate and set the others."
        n2117 = event-data() -> ()  [unwired: 7 out]
        n2118 = property on="Red Laser ON" class="Bool (strict)"("Val(Sgnl)"="Red Laser ON/OFF") -> ()  [unwired: 2 in, 2 out]
        n2119 = property on="Blue Laser ON" class="Bool (strict)"("Val(Sgnl)"="Blue Laser ON/OFF") -> ()  [unwired: 2 in, 2 out]
        n2120 = property on="Green Laser ON" class="Bool (strict)"("Val(Sgnl)"="Green Laser ON/OFF") -> ()  [unwired: 2 in, 2 out]
      }
      event "Laser interlacing mode", "Green Laser ON", "Red Laser ON", "Blue Laser ON": Value Change {
        n2121 = event-data() -> ()  [unwired: 7 out]
        n2122 = local write "Green Laser ON/OFF"("Green Laser ON") -> ()
        n2123 = local write "Blue Laser ON/OFF"("Blue Laser ON") -> ()
        n2124 = local write "Red Laser ON/OFF"("Red Laser ON") -> ()
        n2125 = case shown="True" "Green Laser ON" {
          tunnel: "Laser interlacing mode" -> [_ w3097]
          tunnel: [enum32{"Laser ON", "Laser OFF", "Interlace"}."Laser OFF" ("Green laser mode") w3097] -> w3073
          tunnel: [FALSE w3093] -> w3072
          frame False {
          }
          frame True {
            n2126 = local read "Green FB On/Off"() -> (w3094:bool)
            n2127 = Equal?(x=w3097, y=enum32{"Laser ON", "Laser OFF", "Interlace"}."Interlace") -> (x = y?=w3095:bool)
            n2128 = And(x=w3095, y=w3094) -> (x .and. y?=w3093:bool)
          }
        }
        n2129 = case shown="True" "Red Laser ON" {
          tunnel: "Laser interlacing mode" -> [_ w3090]
          tunnel: [enum32{"Laser ON", "Laser OFF", "Interlace"}."Laser OFF" ("Green laser mode") w3090] -> w3069
          tunnel: [FALSE w3086] -> w3068
          frame False {
          }
          frame True {
            n2130 = local read "Red FB On/Off"() -> (w3087:bool)
            n2131 = Equal?(x=w3090, y=enum32{"Laser ON", "Laser OFF", "Interlace"}."Interlace") -> (x = y?=w3088:bool)
            n2132 = And(x=w3088, y=w3087) -> (x .and. y?=w3086:bool)
          }
        }
        n2133 = case shown="True" "Blue Laser ON" {
          tunnel: "Laser interlacing mode" -> [_ w3081]
          tunnel: [enum32{"Laser ON", "Laser OFF", "Interlace"}."Laser OFF" ("Green laser mode") w3081] -> w3065
          tunnel: [FALSE w3079] -> w3064
          frame False {
          }
          frame True {
            n2134 = local read "Blue FB On/Off"() -> (w3080:bool)
            n2135 = Equal?(x=w3081, y=enum32{"Laser ON", "Laser OFF", "Interlace"}."Interlace") -> (x = y?=w3082:bool)
            n2136 = And(x=w3082, y=w3080) -> (x .and. y?=w3079:bool)
          }
        }
        n2137 = xnode "Read/Write Control"("FPGA VI Reference In"=w3063, "Operating Mode"=w3073, "Operating Mode 2"=w3073, "Green FB On/Off"=w3072, "Red Laser Operating Mode"=w3069, "RI Operating Mode 2"=w3069, "Red FB On/Off"=w3068, "BI Operating Mode (AO)"=w3065, "Blue Laser Operating Mode (D)"=w3065, "Blue FB On/Off"=w3064) -> ("error out"=w3074:errorcluster)  [unwired: 1 in, 1 out]
        n2138 = local read "Red FB On/Off"() -> (w3046:bool)
        n2139 = local read "Green FB On/Off"() -> (w3048:bool)
        n2140 = local read "Green Laser ON"() -> (w3047:bool)
        n2141 = local read "Red Laser ON"() -> (w3045:bool)
        n2142 = And(x=w3046, y=w3045) -> (x .and. y?=w3051:bool)
        n2143 = And(x=w3048, y=w3047) -> (x .and. y?=w3057:bool)
        n2144 = local read "Red laser intensity (V)"() -> (w3050:dbl)
        n2145 = local read "Red FB Setpoint (mV)"() -> (w3049:dbl)
        n2146 = local read "Green FB Setpoint (mV)"() -> (w3060:dbl)
        n2147 = local read "Green laser intensity (V)"() -> (w3062:dbl)
        n2148 = Multiply(x=w3050, y=1000.0) -> (x*y=w3054:dbl)
        n2149 = Subtract(x=w3049, y=5.0) -> (x-y=w3053:dbl)
        n2150 = Multiply(x=w3062, y=1000.0) -> (x*y=w3059:dbl)
        n2151 = Subtract(x=w3060, y=5.0) -> (x-y=w3058:dbl)
        n2152 = Less Or Equal?(x=w3054, y=w3053) -> (x <= y?=w3052:bool)
        n2153 = Less Or Equal?(x=w3059, y=w3058) -> (x <= y?=w3056:bool)
        n2154 = And(x=w3051, y=w3052) -> (x .and. y?=w3041:bool)
        n2155 = And(x=w3057, y=w3056) -> (x .and. y?=w3042:bool)
        n2156 = Or(x=w3042, y=w3041) -> (x .or. y?=w3040:bool)
        n2157 = case shown="True" w3040 {
          frame False {
            n2158 = local write "Laser Intensity Low (bugs to fix)"(FALSE ("Laser Intensity Low")) -> ()
          }
          frame True {
            n2159 = local write "Laser Intensity Low (bugs to fix)"(TRUE ("Laser Intensity Low")) -> ()
          }
        }
      }
      event "Invert laser interlacing", "RF BD 2 to green AOM": Value Change {
        n2160 = event-data() -> ()  [unwired: 7 out]
        n2161 = local read "RF BD 2 to green AOM"() -> (w3098:bool)
        n2162 = xnode "Read/Write Control"("FPGA VI Reference In"=w3099, "Invert GI"="Invert laser interlacing", "Invert GI 2"="Invert laser interlacing", "Invert RI"="Invert laser interlacing", "Invert RI 2"="Invert laser interlacing", "Invert BI (AO)"="Invert laser interlacing", "Invert BI (D)"="Invert laser interlacing", "RF synth bd controls green"=w3098) -> ("error out"=w3101:errorcluster)  [unwired: 1 in, 1 out]
      }
      event "Green FB Setpoint (mV)", "Green FB Gains", "Green FB On/Off", "Green Intensity % (FB OFF)", "Green int current ON count adj": Value Change {
        n2163 = event-data() -> ()  [unwired: 7 out]
        n2164 = local read "Green FB Setpoint (mV)"() -> (w3121:dbl)
        n2165 = Multiply(x=w3121, y=3.2767) -> (x*y=w3105:dbl)
        n2166 = local read "Green Intensity % (FB OFF)"() -> (w3124:dbl)
        n2167 = Multiply(x=w3124, y=655.35) -> (x*y=w3125:dbl)
        n2168 = To Unsigned Word Integer(number=w3125) -> (unsigned 16bit integer=w3123:u16)
        n2169 = local read "Green int current ON count adj"() -> (w3127:u32)
        n2170 = local read "Laser interlacing mode"() -> (w3119:enum32{"Laser ON", "Laser OFF", "Interlace"})
        n2171 = local read "Green FB Gains"() -> (w3116:T11)
        n2172 = local read "Green Laser ON"() -> (w3120:bool)
        n2173 = local read "Green FB On/Off"() -> (w3128:bool)
        n2174 = Equal?(x=w3119, y=enum32{"Laser ON", "Laser OFF", "Interlace"}."Interlace") -> (x = y?=w3117:bool)
        n2175 = Unbundle By Name(w3116) -> ("proportional gain (Kc)"=w3104:i16, "integral gain (Kc*Ts/Ti)"=w3103:i16, "derivative gain (Kc*Td/Ts)"=w3102:i16)
        n2176 = Compound Arithmetic op=AND(w3117, w3128, w3120) -> (w3106:bool)
        n2177 = local read "Green FB Setpoint (mV)"() -> (w3110:dbl)
        n2178 = local read "Green laser intensity (V)"() -> (w3113:dbl)
        n2179 = xnode "Read/Write Control"("FPGA VI Reference In"=w3115, "Green FB Setpoint 2"=w3105, "Green FB Setpoint"=w3105, "Green FB On/Off"=w3106, "Current Out"=w3123, "Green int current ON count adj"=w3127, "P3"=w3104, "I3"=w3103, "D3"=w3102, "P3 2"=w3104, "I3 2"=w3103, "D3 2"=w3102) -> ("error out"=w3129:errorcluster)  [unwired: 1 in, 1 out]
        n2180 = Multiply(x=w3113, y=1000.0) -> (x*y=w3109:dbl)
        n2181 = Subtract(x=w3110, y=5.0) -> (x-y=w3108:dbl)
        n2182 = Less Or Equal?(x=w3109, y=w3108) -> (x <= y?=w3107:bool)
        n2183 = And(x=w3106, y=w3107) -> (x .and. y?=w3114:bool)
        n2184 = case shown="True" w3114 {
          frame False {
            n2185 = local write "Laser Intensity Low (bugs to fix)"(FALSE ("Laser Intensity Low")) -> ()
          }
          frame True {
            n2186 = local write "Laser Intensity Low (bugs to fix)"(TRUE ("Laser Intensity Low")) -> ()
          }
        }
      }
      event "Blue FB Setpoint (mV)", "Blue FB Gains", "Blue FB On/Off", "Blue Intensity % (FB OFF)", "Blue int AO ON count adjust": Value Change {
        # "Triggers blue laser serial command"
        # "16 bit analog out"
        n2187 = event-data() -> ()  [unwired: 7 out]
        n2188 = Multiply(x="Blue FB Setpoint (mV)", y=3.2767) -> (x*y=w3149:dbl)
        n2189 = Multiply(x="Blue Intensity % (FB OFF)", y=0.8) -> (x*y=w3132:dbl)
        n2190 = Number To Decimal String(number=w3132) -> (decimal integer string=w3133:string)  [unwired: 1 in]
        n2191 = Multiply(x="Blue Intensity % (FB OFF)", y=655.35) -> (x*y=w3152:dbl)
        n2192 = local write "Blue Laser Power (mW)\n(Constant Power Mode)"(w3133) -> ()
        n2193 = To Unsigned Word Integer(number=w3152) -> (unsigned 16bit integer=w3151:u16)
        n2194 = local read "Laser interlacing mode"() -> (w3147:enum32{"Laser ON", "Laser OFF", "Interlace"})
        n2195 = Unbundle By Name("Blue FB Gains") -> ("proportional gain (Kc)"=w3144:i16, "integral gain (Kc*Ts/Ti)"=w3143:i16, "derivative gain (Kc*Td/Ts)"=w3142:i16)
        n2196 = local read "Blue Laser ON"() -> (w3137:bool)
        n2197 = Equal?(x=w3147, y=enum32{"Laser ON", "Laser OFF", "Interlace"}."Interlace") -> (x = y?=w3145:bool)
        n2198 = Compound Arithmetic op=AND(w3145, "Blue FB On/Off", w3137) -> (w3148:bool)
        n2199 = xnode "Read/Write Control"("FPGA VI Reference In"=w3136, "Blue FB Setpoint"=w3149, "Blue FB On/Off"=w3148, "BI Current Out"=w3151, "Blue current ON count adj (AO)"="Blue int AO ON count adjust", "P5"=w3144, "I5"=w3143, "D5"=w3142) -> ("error out"=w3154:errorcluster)  [unwired: 1 in, 1 out]
      }
      event "Red FB Setpoint (mV)", "Red FB Gains", "Red FB On/Off", "Red Intensity % (FB OFF)": Value Change {
        n2200 = event-data() -> ()  [unwired: 7 out]
        n2201 = local read "Red FB Setpoint (mV)"() -> (w3175:dbl)
        n2202 = Multiply(x=w3175, y=3.2767) -> (x*y=w3174:dbl)
        n2203 = local read "Red Intensity % (FB OFF)"() -> (w3165:dbl)
        n2204 = Multiply(x=w3165, y=655.35) -> (x*y=w3178:dbl)
        n2205 = To Unsigned Word Integer(number=w3178) -> (unsigned 16bit integer=w3177:u16)
        n2206 = local read "Laser interlacing mode"() -> (w3172:enum32{"Laser ON", "Laser OFF", "Interlace"})
        n2207 = local read "Red FB Gains"() -> (w3169:T11)
        n2208 = local read "Red Laser ON"() -> (w3173:bool)
        n2209 = local read "Red FB On/Off"() -> (w3180:bool)
        n2210 = Equal?(x=w3172, y=enum32{"Laser ON", "Laser OFF", "Interlace"}."Interlace") -> (x = y?=w3170:bool)
        n2211 = Unbundle By Name(w3169) -> ("proportional gain (Kc)"=w3168:i16, "integral gain (Kc*Ts/Ti)"=w3167:i16, "derivative gain (Kc*Td/Ts)"=w3166:i16)
        n2212 = Compound Arithmetic op=AND(w3170, w3180, w3173) -> (w3157:bool)
        n2213 = local read "Red laser intensity (V)"() -> (w3156:dbl)
        n2214 = local read "Red FB Setpoint (mV)"() -> (w3155:dbl)
        n2215 = xnode "Read/Write Control"("FPGA VI Reference In"=w3164, "Red FB Setpoint"=w3174, "Red FB On/Off"=w3157, "RI Current Out"=w3177, "P4"=w3168, "I4"=w3167, "D4"=w3166) -> ("error out"=w3181:errorcluster)  [unwired: 1 in, 1 out]
        n2216 = Multiply(x=w3156, y=1000.0) -> (x*y=w3161:dbl)
        n2217 = Subtract(x=w3155, y=5.0) -> (x-y=w3160:dbl)
        n2218 = Less Or Equal?(x=w3161, y=w3160) -> (x <= y?=w3159:bool)
        n2219 = And(x=w3157, y=w3159) -> (x .and. y?=w3158:bool)
        n2220 = case shown="False" w3158 {
          frame False {
            n2221 = local write "Laser Intensity Low (bugs to fix)"(FALSE ("Laser Intensity Low")) -> ()
          }
          frame True {
            n2222 = local write "Laser Intensity Low (bugs to fix)"(TRUE ("Laser Intensity Low")) -> ()
          }
        }
      }
      event "+ phase (APD 1 Gate)", "- phase (APD 1 Gate)", "+ phase (APD 2 Gate)", "- phase (APD 2 Gate)", "+ phase (APD 3 Gate)", "- phase (APD 3 Gate)", "+ phase (APD Acq)", "- phase (APD Acq)": Value Change {
        n2223 = event-data() -> ()  [unwired: 7 out]
        n2224 = local read "Phase Adj. (APD 1 Gate)"() -> (w3204:i16)
        n2225 = Or(x="- phase (APD 1 Gate)", y="+ phase (APD 1 Gate)") -> (x .or. y?=w3206:bool)
        n2226 = Negate(x=w3204) -> (-x=w3211:i16)
        n2227 = Select(t=w3211, s="+ phase (APD 1 Gate)", f=w3204) -> (s? t:f=w3210:i16)
        n2228 = local read "Phase Adj. (APD 2 Gate)"() -> (w3201:i16)
        n2229 = Or(x="- phase (APD 2 Gate)", y="+ phase (APD 2 Gate)") -> (x .or. y?=w3199:bool)
        n2230 = Negate(x=w3201) -> (-x=w3203:i16)
        n2231 = Select(t=w3203, s="+ phase (APD 2 Gate)", f=w3201) -> (s? t:f=w3200:i16)
        n2232 = Negate(x="Phase Adj. (APD 3 Gate)") -> (-x=w3198:i16)
        n2233 = Or(x="- phase (APD 3 Gate)", y="+ phase (APD 3 Gate)") -> (x .or. y?=w3194:bool)
        n2234 = Select(t=w3198, s="+ phase (APD 3 Gate)", f="Phase Adj. (APD 3 Gate)") -> (s? t:f=w3195:i16)
        n2235 = local read "Phase Adj. (APD Acq)"() -> (w3192:i16)
        n2236 = Or(x="- phase (APD Acq)", y="+ phase (APD Acq)") -> (x .or. y?=w3190:bool)
        n2237 = Negate(x=w3192) -> (-x=w3193:i16)
        n2238 = Select(t=w3193, s="+ phase (APD Acq)", f=w3192) -> (s? t:f=w3191:i16)
        n2239 = xnode "Read/Write Control"("FPGA VI Reference In"=w3184, "Phase count adjustment (APD 1 Gate)"=w3210, "Phase count adjustment (APD 2 Gate)"=w3200, "Phase count adjustment (APD 3 Gate)"=w3195, "Phase Count Adjustment (APD Acq)"=w3191) -> ("FPGA VI Reference Out"=w3208:T25, "error out"=w3209:errorcluster)  [unwired: 1 in]
        n2240 = xnode "Read/Write Control"("FPGA VI Reference In"=w3208, "error in"=w3209, "+ phase (APD 1 Gate)"=w3206, "+ phase (APD 2 Gate)"=w3199, "+ phase (APD 3 Gate)"=w3194, "+ phase (APD Acq)"=w3190) -> ("error out"=w3207:errorcluster)  [unwired: 1 out]
      }
      event "Invert APD Gate", "APD Gate ON Count", "APD Gate OFF Count", "APD Gate", "APD Integration Time (s)", "APD AO Scale Factor", "Duty Frequency (ON 1/N cycles)", "Interlace ON count", "Interlace OFF count", "APD host processing integration": Value Change {
        n2241 = event-data() -> ()  [unwired: 7 out]
        n2242 = Add(x="Interlace ON count", y="Interlace OFF count") -> (x+y=w3222:u16)
        n2243 = Add(x="APD Gate ON Count", y="APD Gate OFF Count") -> (x+y=w3232:u16)
        n2244 = Multiply(x="APD Integration Time (s)", y="APD host processing integration") -> (x*y=→"Host fluorescence integration time (s)":dbl)
        n2245 = Multiply(x="Duty Frequency (ON 1/N cycles)", y=w3222) -> (x*y=w3218:u16)
        "Green AI Count" <- w3218
        "Red AI Count" <- w3218
        "Blue AI Count" <- w3218
        n2246 = Subtract(x=w3218, y="Interlace ON count") -> (x-y=w3221:u16)
        n2247 = Multiply(x=w3232, y="Duty Frequency (ON 1/N cycles)") -> (x*y=w3231:u16)
        n2248 = Subtract(x=w3231, y="APD Gate ON Count") -> (x-y=w3230:u16)
        n2249 = Reciprocal(x="APD Integration Time (s)") -> (1/x=→"APD Acq Rate (Hz)":dbl)
        n2250 = local read "DMA Update Period (s)"() -> (w3233:dbl)
        n2251 = Multiply(x="APD Integration Time (s)", y=40000000.0) -> (x*y=w3236:dbl)
        n2252 = To Unsigned Long Integer(number=w3236) -> (unsigned 32bit integer=w3224:u32)
        "APD Int. Count" <- w3224
        n2253 = local read "Number of APDs"() -> (w3217:u8)
        n2254 = Divide(x=w3233, y="APD Integration Time (s)") -> (x/y=w3212:dbl)
        n2255 = Multiply(x=w3217, y=w3212) -> (x*y=w3234:dbl)
        n2256 = property on="APD Samples/FIFO Acq." class="DigNum (strict)"("Val(Sgnl)"=w3212) -> ()  [unwired: 2 in, 2 out]
        n2257 = local write "APD Elements/DMA read"(w3234) -> ()
        n2258 = xnode "Read/Write Control"("FPGA VI Reference In"=w3216, "Invert APD Gate"="Invert APD Gate", "APD Gate ON Count"="APD Gate ON Count", "APD Gate OFF Count"=w3230, "APD Acq Rate Count"=w3224, "APD Gate Operating Mode"="APD Gate", "APD AO scale factor"="APD AO Scale Factor", "Green interlace ON count"="Interlace ON count", "Green interlace OFF count"=w3221, "Green interlace ON count 2"="Interlace ON count", "Green interlace OFF count 2"=w3221, "Green FB Count"=w3218, "Red interlace ON count"="Interlace ON count", "Red interlace OFF count"="Interlace OFF count", "Blue ON count (AO)"="Interlace ON count", "Blue OFF count (AO)"="Interlace OFF count", "Blue interlace OFF count (D)"="Interlace OFF count", "Blue interlace ON count (D)"="Interlace ON count") -> ("error out"=w3238:errorcluster)  [unwired: 1 in, 1 out]
      }
      event "ALEX green on count", "ALEX red on count", "ALEX ON": Value Change {
        n2259 = event-data() -> ()  [unwired: 7 out]
        n2260 = local read "ALEX green on count"() -> (w3241:i16)
        n2261 = local read "ALEX red on count"() -> (w3240:i16)
        n2262 = xnode "Read/Write Control"("FPGA VI Reference In"=w3242, "ALEX green on count"=w3241, "ALEX red on count"=w3240, "ALEX ON"="ALEX ON") -> ()  [unwired: 1 in, 2 out]
      }
      event "Lifetime timeout (APD1)": Value Change {
        n2263 = event-data() -> ()  [unwired: 7 out]
        n2264 = Multiply(x="Lifetime timeout (APD1)", y=0.005) -> (x*y=→"Lifetime timeout APD1 (us)":dbl)
        n2265 = xnode "Read/Write Control"("FPGA VI Reference In"=w3246, "Lifetime timeout APD1"="Lifetime timeout (APD1)") -> ()  [unwired: 1 in, 2 out]
      }
      event "Neg. TTrig FPGA": Value Change {
        n2266 = event-data() -> ()  [unwired: 7 out]
        n2267 = xnode "Read/Write Control"("FPGA VI Reference In"=w3247, "TTrig Negate Pos"="Neg. TTrig FPGA") -> ()  [unwired: 1 in, 2 out]
      }
      event "Test ttrig": Value Change {
        n2268 = event-data() -> ()  [unwired: 7 out]
        n2269 = xnode "Read/Write Control"("FPGA VI Reference In"=w3249, "TTrig?"=TRUE) -> ("error out"=w3251:errorcluster)  [unwired: 1 in, 1 out]
      }
      event "Number of F/B Scans (AOD)", "Scan Speed (nm/s)", "Scan BD", "Initial delta (MHz)", "Step Size (nm)", "Scan Range (nm)": Value Change {
        w3315 = 123.0  # AOM cal (nm/MHz)
        n2270 = event-data() -> ()  [unwired: 7 out]
        n2271 = local read "BD 1 Frequency 1 (MHz)"() -> (w3298:dbl)
        n2272 = local read "AOM X Cal (nm/MHz)"() -> (w3290:dbl)
        n2273 = local read "X RF Frequency Limits (MHz)"() -> (w3302:T18)
        n2274 = local read "Y RF Frequency Limits (MHz)"() -> (w3299:T18)
        n2275 = local read "BD 2 Frequency 1 (MHz)"() -> (w3304:dbl)
        n2276 = Negate(x="Scan Range (nm)") -> (-x=w3268:dbl)
        n2277 = Divide(x=w3268, y=w3290) -> (x/y=w3272:dbl)
        n2278 = Select(t=w3302, s="Scan BD", f=w3299) -> (s? t:f=w3301:T18)
        n2279 = Select(t=w3298, s="Scan BD", f=w3304) -> (s? t:f=w3303:dbl)
        n2280 = Unbundle By Name(w3301) -> ("Maximum"=w3310:dbl, "Minimum"=w3309:dbl)
        n2281 = Add(x=w3272, y=w3303) -> (x+y=w3307:dbl)
        n2282 = Divide(x=w3268, y="Step Size (nm)") -> (x/y=w3287:dbl)
        n2283 = Divide(x="Step Size (nm)", y=w3290) -> (x/y=w3296:dbl)
        n2284 = Absolute Value(x=w3287) -> (abs(x)=w3271:dbl)
        n2285 = Sign(1:w3268) -> (0:w3269:dbl)
        n2286 = In Range and Coerce(upper limit=w3310, x=w3307, lower limit=w3309) -> (coerced(x)=w3306:dbl, In Range?=w3308:bool)
        n2287 = To Unsigned Quad Integer(1:w3271) -> (0:w3286:u64)
        "Scan steps (AOD)" <- w3286
        n2288 = call "IR AOM freq to word.vi"("Frequency In (MHz)"=w3296) -> ("Frequency Word Out (double)"=w3293:dbl)
        n2289 = Multiply(x=w3269, y=w3293) -> (x*y=w3270:dbl)
        n2290 = Subtract(x=w3307, y=w3306) -> (x-y=w3305:dbl)
        n2291 = To Quad Integer(1:w3270) -> (0:w3292:i64)
        "Incr. int (AOD)" <- w3292
        n2292 = Subtract(x=w3272, y=w3305) -> (x-y=w3291:dbl)
        "Scan Range (MHz)" <- w3291
        n2293 = Select(t=w3272, s=w3308, f=w3291) -> (s? t:f=w3311:dbl)
        n2294 = Multiply(x=w3291, y=w3290) -> (x*y=w3289:dbl)
        n2295 = Decrement(x=w3286) -> (x-1=w3339:u64)
